vi "梦幻城堡C1~3通信.vi"() -> ()   [LabVIEW 2016, in "环境动力监测库.lvlib" / "UPS库.lvlib"]
uses:
  <vilib>/Instr/_visa.llb/VISA Configure Serial Port (Instr).vi
  <vilib>/Utility/config.llb/NI_LVConfig.lvlib
panel:
  out "Status":T1
  in  "open":bool
  in  "close":bool
  out "通信指示":bool
  in  "关机":bool
  in  "状态查询":bool
  out "读取缓冲区":string
  # "输入电压"
  # "输入故障电压"
  # "输出电压"
  # "输出电流百分比"
  # "输入频率"
  # "电池电压"
  # "UPS温度"
  # "UPS状态"
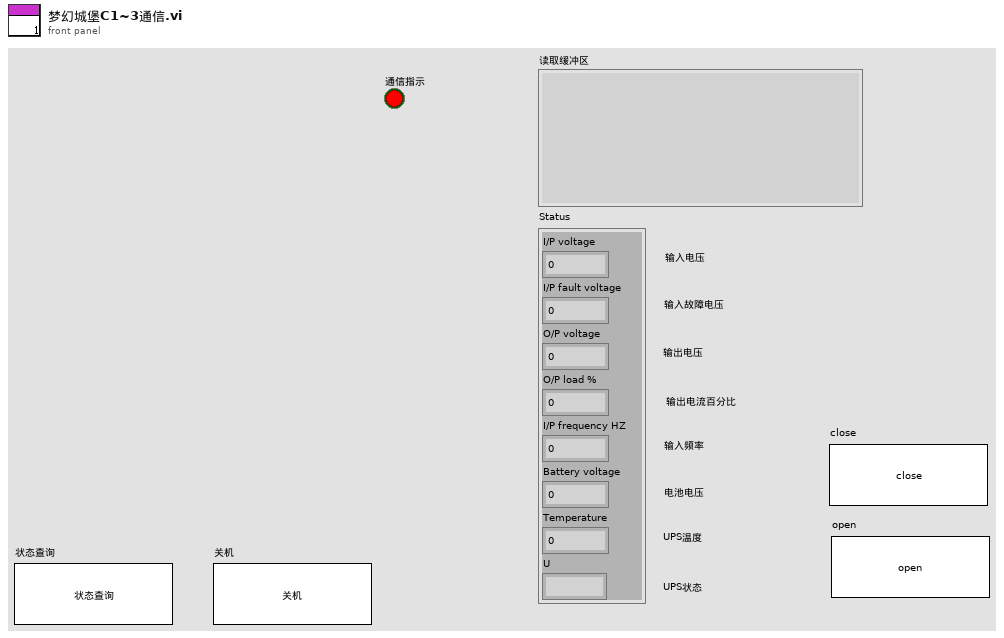
[diagram p1: front panel]
types:
  T1 = cluster{"I/P voltage":dbl, "I/P fault voltage":dbl, "O/P voltage":dbl, "O/P load %":dbl, "I/P frequency HZ":dbl, "Battery voltage":dbl, "Temperature":dbl, "U":string}
  T2 = cluster{"枚举":enum16{"open", "read", "write", "close"}, "写入缓冲区":string}
  T3 = typedef "NI_LVConfig.lvlib/Config Data RefNum.ctl" = refnum<k1>
  T4 = cluster{"baud rate (9600)":u32, "stop bits (10: 1 bit)":u16, "parity (0:none)":enum16{"None", "Odd", "Even", "Mark", "Space"}, "data bits (8)":u16, "timeout (10sec)":u32}
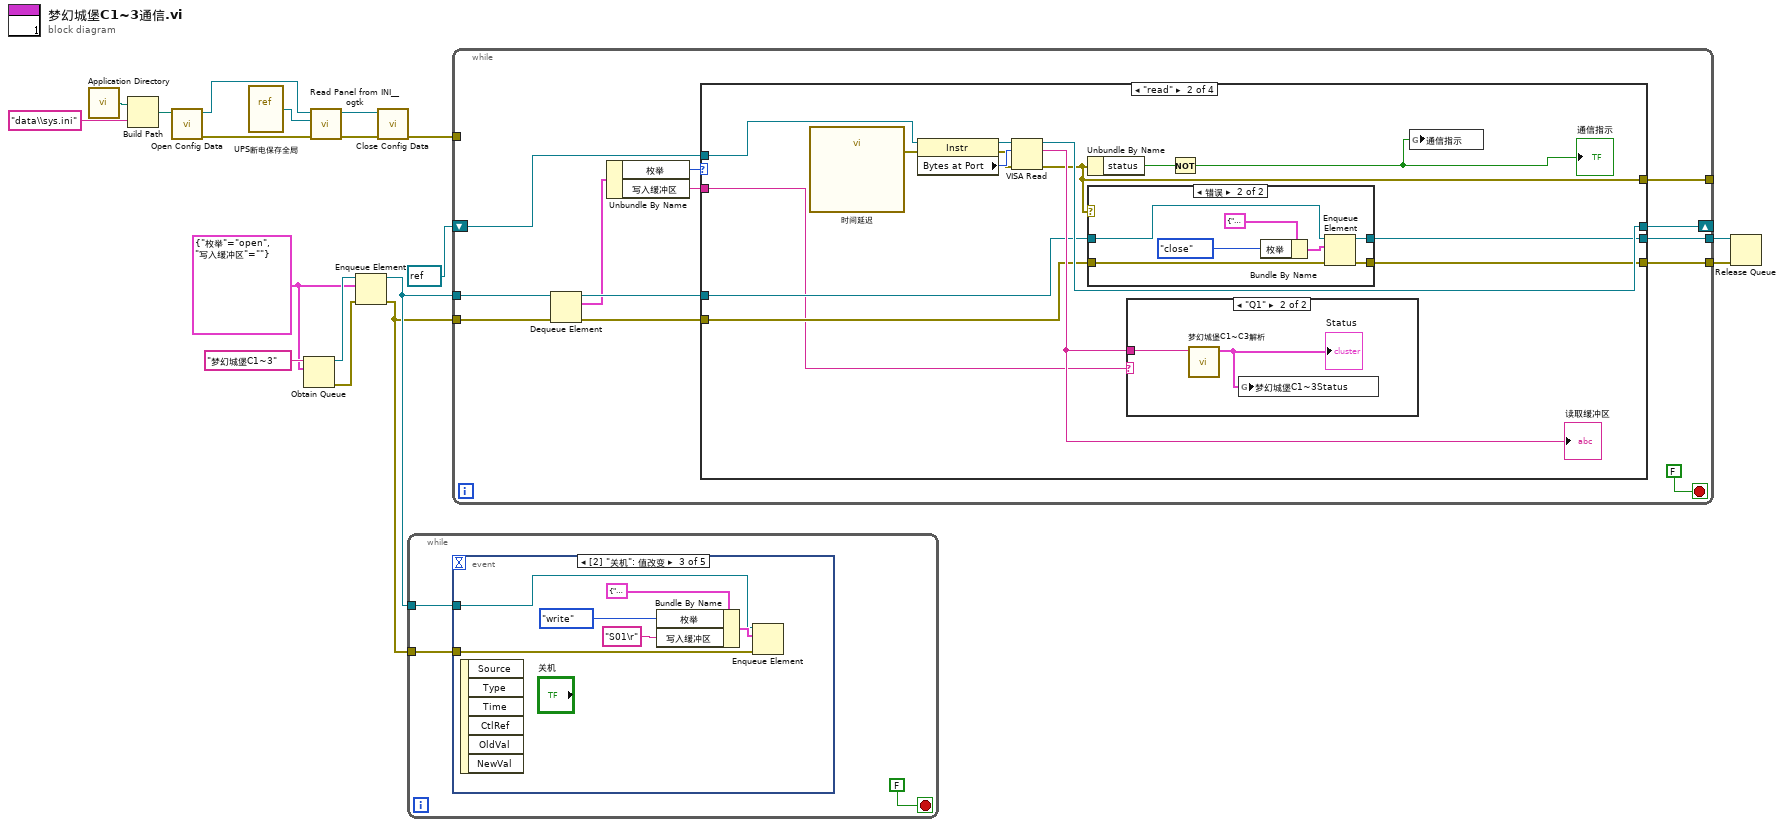
[diagram p0: block diagram]
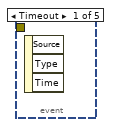
[diagram p2: hidden frame]
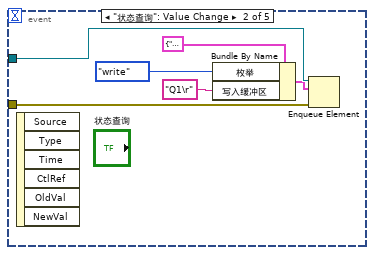
[diagram p3: hidden frame]
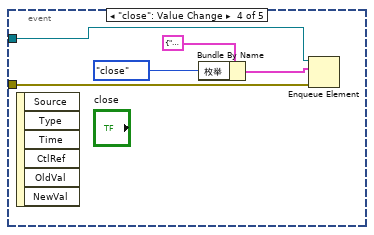
[diagram p4: hidden frame]
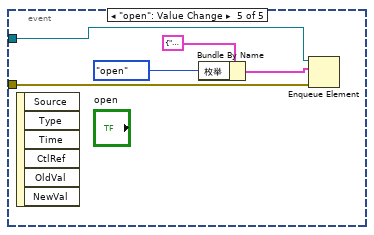
[diagram p5: hidden frame]
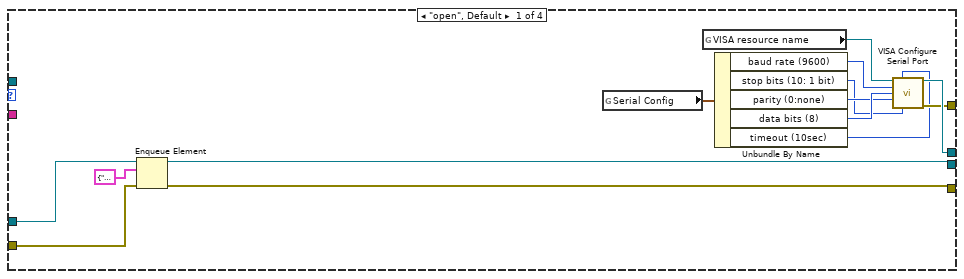
[diagram p6: hidden frame]
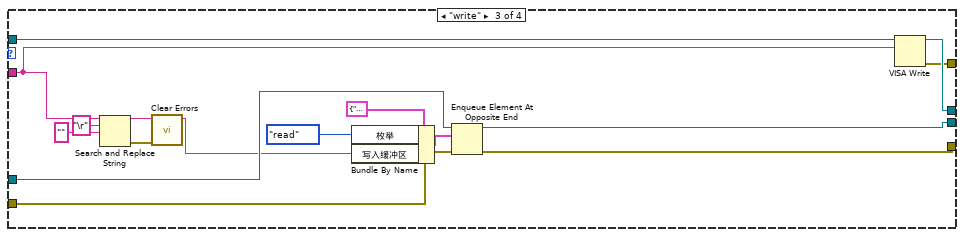
[diagram p9: hidden frame]
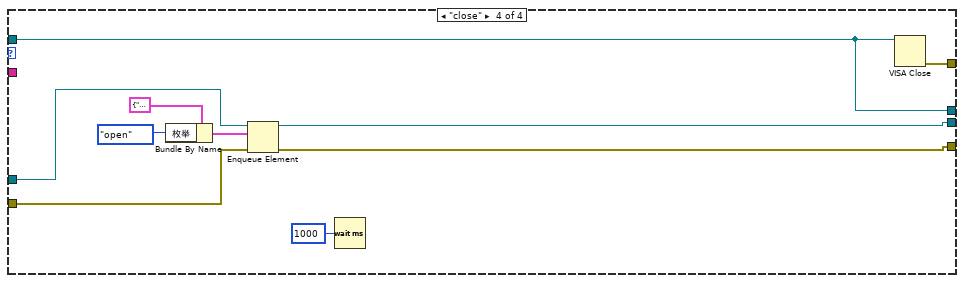
[diagram p10: hidden frame]
diagram:
  w12 = T2 {"枚举"=enum."open", "写入缓冲区"=""}
  n1 = call <vilib>:"Application Directory.vi"() -> ("Application Directory"=w9:path)
  n2 = Build Path(base path=w9, name or relative path="data\\sys.ini" ("名称或相对路径")) -> (appended path=w7:path)
  n3 = call <vilib>:"Open Config Data.vi"("configuration file path"=w7) -> ("error out"=w3:errorcluster, "refnum"=w6:T3)  [unwired: 8 in, 1 out]
  n4 = vi-ref "UPS断电保存全局.vi"() -> (w5:refnum<vi>)
  n5 = Obtain Queue(name (unnamed)="梦幻城堡C1~3" ("名称（未命名）"), element data type=w12) -> (queue out=w17:refnum<queue>, error out=w16:errorcluster)  [unwired: 3 in, 1 out]
  n6 = call <userlib>:"Read Panel from INI__ogtk.vi"("error in (no error)"=w3, "VI ref"=w5, "refnum"=w6) -> ("error out"=w2:errorcluster, "refnum out"=w4:T3)  [unwired: 7 in]
  n7 = Enqueue Element(queue=w17, element=w12, error in (no error)=w16) -> (queue out=w15:refnum<queue>, error out=w14:errorcluster)  [unwired: 1 in, 1 out]
  n8 = call <vilib>:"Close Config Data.vi"("error in (no error)"=w2, "refnum"=w4) -> ("error out"=w1:errorcluster)  [unwired: 8 in, 1 out]
  n9 = while {
    tunnel: w15 -> [w20]
    tunnel: w14 -> [w19]
    stop <- FALSE stop-if-true
    n10 = event shown="[2] \"关机\": 值改变" {
      selector: _ -> [_ _ _ _ _]
      dyn-events: _ -> [_ _ _ _ _]
      timeout: _ -> [_ _ _ _ _]
      tunnel: w20 -> [_ w26 w30 w38 w43]
      tunnel: w19 -> [_ w22 w29 w37 w42]
      event Timeout {
        n11 = event-data() -> ()  [unwired: 1 in, 3 out]
      }
      event "状态查询": Value Change {
        n12 = event-data() -> ()  [unwired: 1 in, 6 out]
        n13 = Bundle By Name(cluster=T2 {"枚举"=enum."open", "写入缓冲区"=""}, "枚举"=enum16{"open", "read", "write", "close"}."write" ("元素"), "写入缓冲区"="Q1\r") -> (w25:T2)
        n14 = Enqueue Element(queue=w26, element=w25, error in (no error)=w22) -> ()  [unwired: 1 in, 3 out]
      }
      event "关机": Value Change {
        n15 = event-data() -> ()  [unwired: 1 in, 6 out]
        n16 = Bundle By Name(cluster=T2 {"枚举"=enum."open", "写入缓冲区"=""}, "枚举"=enum16{"open", "read", "write", "close"}."write" ("元素"), "写入缓冲区"="S01\r") -> (w32:T2)
        n17 = Enqueue Element(queue=w30, element=w32, error in (no error)=w29) -> ()  [unwired: 1 in, 3 out]
      }
      event "close": Value Change {
        n18 = event-data() -> ()  [unwired: 1 in, 6 out]
        n19 = Bundle By Name(cluster=T2 {"枚举"=enum."open", "写入缓冲区"=""}, "枚举"=enum16{"open", "read", "write", "close"}."close") -> (w34:T2)
        n20 = Enqueue Element(queue=w38, element=w34, error in (no error)=w37) -> ()  [unwired: 1 in, 3 out]
      }
      event "open": Value Change {
        n21 = event-data() -> ()  [unwired: 1 in, 6 out]
        n22 = Bundle By Name(cluster=T2 {"枚举"=enum."open", "写入缓冲区"=""}, "枚举"=enum16{"open", "read", "write", "close"}."open") -> (w39:T2)
        n23 = Enqueue Element(queue=w43, element=w39, error in (no error)=w42) -> ()  [unwired: 1 in, 3 out]
      }
    }
  }
  n24 = while {
    shift-right: [w56] -> _
    shift-left: refnum<visa-resource-name> refnum ("VISA resource name out") -> [w55]
    tunnel: [w54] -> _
    tunnel: w15 -> [w52]
    tunnel: w14 -> [w51]
    tunnel: [w47] -> w10
    tunnel: [w48] -> w11
    tunnel: w1 -> [_]
    stop <- FALSE stop-if-true
    n25 = Dequeue Element(queue=w52, error in (no error)=w51) -> (queue out=w50:refnum<queue>, element=w46:T2, error out=w49:errorcluster)  [unwired: 1 in, 1 out]
    n26 = Unbundle By Name(w46) -> ("枚举"=w45:enum16{"open", "read", "write", "close"}, "写入缓冲区"=w44:string)
    n27 = case shown="\"read\"" w45 {
      tunnel: [w70 w82 w110 w120] -> w56
      tunnel: w55 -> [_ w85 w111 w120]
      tunnel: [w69 w78 w109 w121] -> w54
      tunnel: w50 -> [w61 w77 w108 w116]
      tunnel: w49 -> [w60 w76 w107 w115]
      tunnel: [w59 w75 w103 w114] -> w48
      tunnel: [w58 w74 w102 w113] -> w47
      tunnel: w44 -> [_ w72 w101 _]
      frame "open", Default {
        n28 = Enqueue Element(queue=w61, element=T2 {"枚举"=enum."read", "写入缓冲区"=""}, error in (no error)=w60) -> (queue out=w59:refnum<queue>, error out=w58:errorcluster)  [unwired: 1 in, 1 out]
        n29 = global read "UPS断电保存全局.vi" "Serial Config"() -> (w67:T4)
        n30 = global read "UPS断电保存全局.vi" "VISA resource name"() -> (w68:refnum<visa-resource-name>)
        n31 = Unbundle By Name(w67) -> ("baud rate (9600)"=w66:u32, "stop bits (10: 1 bit)"=w63:u16, "parity (0:none)"=w64:enum16{"None", "Odd", "Even", "Mark", "Space"}, "data bits (8)"=w65:u16, "timeout (10sec)"=w62:u32)
        n32 = call-poly "VISA Configure Serial Port"("VISA resource name"=w68, "timeout (10sec)"=w62, "baud rate (9600)"=w66, "data bits (8)"=w65, "parity (0:none)"=w64, "stop bits (10: 1 bit)"=w63) -> ("VISA resource name out"=w70:refnum<visa-resource-name>, "error out"=w69:errorcluster)  [unwired: 8 in]
      }
      frame "read" {
        n33 = call "时间延迟"() -> ("error out"=w80:errorcluster)  [unwired: 11 in]
        n34 = property class="Instr"(reference=w85, error in=w80) -> (reference out=w83:refnum<visa-resource-name>, error out=w71:errorcluster, "Bytes at Port"=w84:u32)
        n35 = VISA Read(VISA resource name=w83, byte count=w84, error in (no error)=w71) -> (VISA resource name out=w82:refnum<visa-resource-name>, read buffer=w79:string, error out=w78:errorcluster)  [unwired: 1 out]
        "读取缓冲区" <- w79
        n36 = Unbundle By Name(w78) -> ("status"=w81:bool)
        n37 = case shown="错误" w78 {
          tunnel: w77 -> [w89 w90]
          tunnel: w76 -> [w88 w93]
          tunnel: [w89 w92] -> w75
          tunnel: [w88 w91] -> w74
          frame No Error {
          }
          frame Error {
            n38 = Bundle By Name(cluster=T2 {"枚举"=enum."open", "写入缓冲区"=""}, "枚举"=enum16{"open", "read", "write", "close"}."close") -> (w95:T2)
            n39 = Enqueue Element(queue=w90, element=w95, error in (no error)=w93) -> (queue out=w92:refnum<queue>, error out=w91:errorcluster)  [unwired: 1 in, 1 out]
          }
        }
        n40 = case shown="\"Q1\"" w72 {
          tunnel: w79 -> [_ w86]
          frame "假", Default {
          }
          frame "Q1" {
            n41 = call "梦幻城堡C1~C3解析.vi"("读取缓冲区"=w86) -> ("Status"=w87:T1)  [unwired: 10 in]
            "Status" <- w87
            n42 = global write "UPS内部交互全局.vi" "梦幻城堡C1~3Status"(w87) -> ()
          }
        }
        n43 = Not(x=w81) -> (.not. x?=w73:bool)
        "通信指示" <- w73
        n44 = global write "UPS内部交互全局.vi" "通信指示"(w73) -> ()
      }
      frame "write" {
        n45 = Search and Replace String(input string=w101, search string="\r" ("搜索字符串"), replace string="" ("替换字符串(\"\")")) -> (result string=w98:string, error out=w97:errorcluster)  [unwired: 5 in, 2 out]
        n46 = call <vilib>:"Clear Errors.vi"("error in (no error)"=w97) -> ()  [unwired: 5 in, 2 out]
        n47 = Bundle By Name(cluster=T2 {"枚举"=enum."open", "写入缓冲区"=""}, "枚举"=enum16{"open", "read", "write", "close"}."read", "写入缓冲区"=w98) -> (w104:T2)
        n48 = Enqueue Element At Opposite End(queue=w108, element=w104, error in (no error)=w107) -> (queue out=w103:refnum<queue>, error out=w102:errorcluster)  [unwired: 1 in, 1 out]
        n49 = VISA Write(VISA resource name=w111, write buffer=w101) -> (VISA resource name out=w110:refnum<visa-resource-name>, error out=w109:errorcluster)  [unwired: 1 in, 1 out]
      }
      frame "close" {
        n50 = Bundle By Name(cluster=T2 {"枚举"=enum."open", "写入缓冲区"=""}, "枚举"=enum16{"open", "read", "write", "close"}."open") -> (w117:T2)
        n51 = Enqueue Element(queue=w116, element=w117, error in (no error)=w115) -> (queue out=w114:refnum<queue>, error out=w113:errorcluster)  [unwired: 1 in, 1 out]
        n52 = Wait (ms)(milliseconds to wait=u32 1000 ("等待时间（毫秒）")) -> ()  [unwired: 1 out]
        n53 = VISA Close(VISA resource name=w120) -> (error out=w121:errorcluster)  [unwired: 1 in]
      }
    }
  }
  n54 = Release Queue(queue=w11, error in (no error)=w10) -> ()  [unwired: 1 in, 3 out]
